vi "Remove Recieved Test From Running List.vi"(8 "Finished Test":path, 11 "Running Tests in":T1) -> (3 "Running Tests out":T1)   [LabVIEW 2011]
uses:
  Controls/ListBox Test Record.ctl
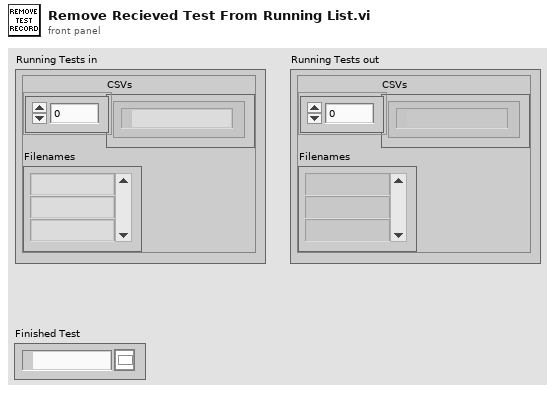
[diagram p1: front panel]
types:
  T1 = typedef "ListBox Test Record.ctl" = cluster{"CSVs":path[], "Filenames":string[]}
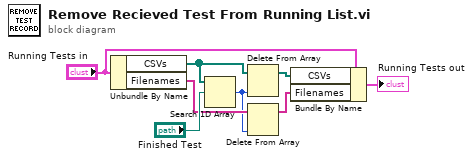
[diagram p0: block diagram]
diagram:
  n1 = Unbundle By Name("Running Tests in") -> ("CSVs"=w7:path[], "Filenames"=w6:string[])
  n2 = Search 1D Array(1D array=w7, element="Finished Test") -> (index of element=w5:i32)  [unwired: 1 in]
  n3 = Delete From Array(array=w7, index=w5) -> (array with subset deleted=w3:path[])  [unwired: 1 in, 1 out]
  n4 = Delete From Array(array=w6, index=w5) -> (array with subset deleted=w2:string[])  [unwired: 1 in, 1 out]
  n5 = Bundle By Name(cluster="Running Tests in", "CSVs"=w3, "Filenames"=w2) -> (→"Running Tests out":T1)
